vi "G#Object_GetAggregatedObjects.vi"(0 "reference in":refnum<class "G#Object.lvclass">, 2 "class attributes (F)":bool, 3 "array names (T)":bool=TRUE, 4 "remove duplicates (F)":bool, 5 "error in (no error)":errorcluster) -> (14 "reference out":refnum<class "G#Object.lvclass">, 15 "aggregated objects":refnum<class "G#Object.lvclass">[](array[class]), 16 "aggregated names":string[](array[string]), 19 "error out":errorcluster)   [LabVIEW 2020, in "G#Object.lvclass"]
doc: "Returns the aggregated objects (references in the object attributes) for the specified objects."
uses:
  <vilib>/addons/_AddQ/G#Object/G#Object.lvclass
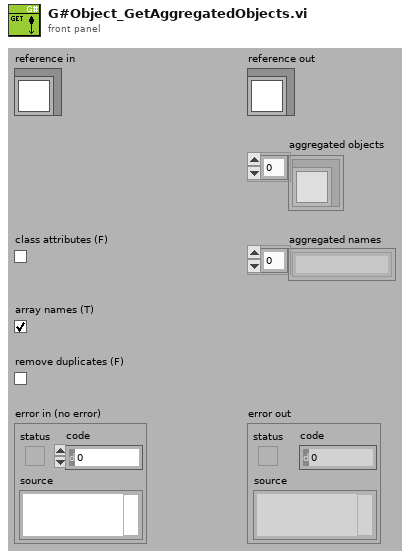
[diagram p1: front panel]
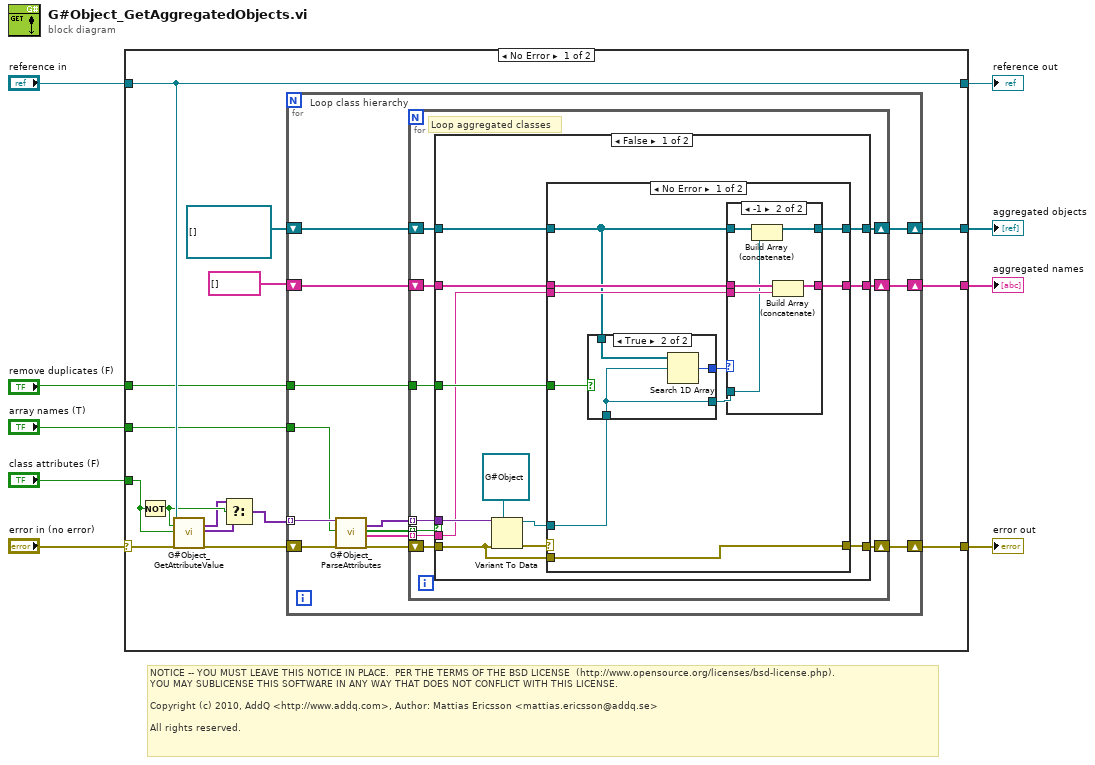
[diagram p0: block diagram]
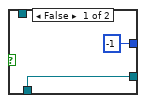
[diagram p2: hidden frame]
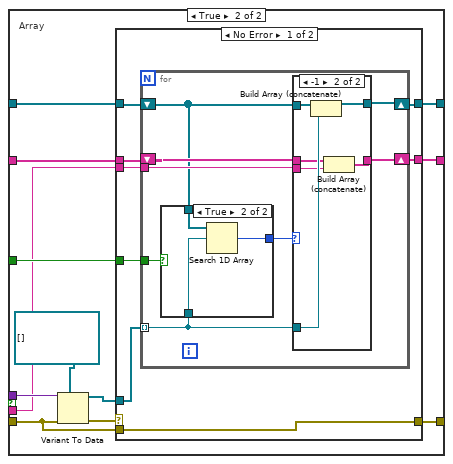
[diagram p5: hidden frame]
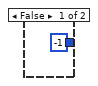
[diagram p6: hidden frame]
diagram:
  # "NOTICE -- YOU MUST LEAVE THIS NOTICE IN PLACE.  PER THE TERMS OF THE BSD LICENSE  (http://www.opensource.org/licenses/bsd-license.php).\nYOU MAY SUBLICENSE THIS SOFTWARE IN ANY WAY THAT DOES NOT CONFLICT WITH THIS LICENSE.\n\nCopyright (c) 2010, AddQ <http://www.addq.com>, Author: Mattias Ericsson <mattias.ericsson@addq.se>\n\nAll rights reserved."
  n1 = case shown="No Error" "error in (no error)" {
    selector: "error in (no error)" -> [w24 w130]
    tunnel: [w20 w130] -> w8
    tunnel: [w23 w129] -> w6
    tunnel: "reference in" -> [w23 w129]
    tunnel: [w19 _] -> w5
    tunnel: "class attributes (F)" -> [w18 _]
    tunnel: "remove duplicates (F)" -> [w13 _]
    tunnel: [w11 _] -> w2
    tunnel: "array names (T)" -> [w10 _]
    frame No Error {
      n2 = Not(x=w18) -> (.not. x?=w17:bool)
      n3 = call <vilib>:"G#Object_GetAttributeValue.vi"("reference in"=w23, "object attributes (T)"=w17, "class attributes (F)"=w18, "error in (no error)"=w24) -> ("attributes"=w16:variant[], "class attributes"=w15:variant[], "error out"=w22:errorcluster)  [unwired: 11 in, 2 out]
      n4 = Select(t=w16, s=w17, f=w15) -> (s? t:f=w14:variant[])
      n5 = for {
        shift-right: [w31] -> w20
        shift-left: w22 -> [w37]
        tunnel: w14 -> [w29] mode=indexing
        shift-right: [w32] -> w19
        shift-left: refnum<class "G#Object.lvclass">[] [] ("aggregated objects") -> [w33]
        tunnel: w13 -> [w30]
        shift-right: [w26] -> w11
        shift-left: string[] [] ("AttributeName") -> [w28]
        tunnel: w10 -> [w25]
        # "Loop class hierarchy"
        n6 = call <vilib>:"G#Object_ParseAttributes.vi"("attributes"=w29, "array names (T)"=w25, "error in (no error)"=w37) -> ("LabVIEWClassElements"=w35:variant[], "array?"=w34:bool[], "attribute name"=w27:string[], "error out"=w36:errorcluster)  [unwired: 13 in]
        n7 = for {
          shift-right: [w42] -> w31
          shift-left: w36 -> [w46]
          tunnel: w35 -> [w45] mode=indexing
          tunnel: w34 -> [w47] mode=indexing
          shift-right: [w43] -> w32
          shift-left: w33 -> [w44]
          tunnel: w30 -> [w41]
          shift-right: [w38] -> w26
          shift-left: w28 -> [w40]
          tunnel: w27 -> [w39] mode=indexing
          # "Loop aggregated classes"
          n8 = case shown="False" w47 {
            tunnel: w46 -> [w52 w91]
            tunnel: w45 -> [w59 w97]
            tunnel: w44 -> [w56 w95]
            tunnel: [w54 w94] -> w42
            tunnel: [w53 w93] -> w43
            tunnel: w41 -> [w51 w89]
            tunnel: w40 -> [w50 w88]
            tunnel: w39 -> [w49 w86]
            tunnel: [w48 w87] -> w38
            frame False {
              n9 = Variant To Data(error in=w52, type=refnum<class "G#Object.lvclass"> refnum ("G#Object.lvclass"), Variant=w59) -> (data=w55:refnum<class "G#Object.lvclass">, error out=w57:errorcluster)
              n10 = case shown="No Error" w57 {
                tunnel: w56 -> [w61 w85]
                tunnel: w55 -> [w67 _]
                tunnel: [w68 w84] -> w54
                tunnel: [w69 w85] -> w53
                tunnel: w52 -> [w68 w84]
                tunnel: w51 -> [w65 _]
                tunnel: w50 -> [w64 w83]
                tunnel: w49 -> [w63 _]
                tunnel: [w62 w83] -> w48
                frame No Error {
                  n11 = case shown="True" w65 {
                    tunnel: w67 -> [w70 w72]
                    tunnel: [-1 ("index of element") w74] -> w66
                    tunnel: w61 -> [_ w73]
                    tunnel: [w70 w72] -> w60
                    frame False {
                    }
                    frame True {
                      n12 = Search 1D Array(1D array=w73, element=w72) -> (index of element=w74:i32)  [unwired: 1 in]
                    }
                  }
                  n13 = case shown="-1" w66 {
                    tunnel: w61 -> [w76 w82]
                    tunnel: [w76 w81] -> w69
                    tunnel: w64 -> [w75 w80]
                    tunnel: w63 -> [_ w79]
                    tunnel: [w75 w78] -> w62
                    tunnel: w60 -> [_ w77]
                    frame Default {
                      # "Already\nadded"
                    }
                    frame -1 {
                      n14 = Build Array (concatenate)(w82, w77) -> (w81:refnum<class "G#Object.lvclass">[])
                      n15 = Build Array (concatenate)(w80, w79) -> (w78:string[])
                    }
                  }
                }
                frame Error {
                  # "Not a G# Object"
                }
              }
            }
            frame True {
              # "Array"
              n16 = Variant To Data(error in=w91, type=refnum<class "G#Object.lvclass">[] [] ("aggregated objects"), Variant=w97) -> (data=w90:refnum<class "G#Object.lvclass">[], error out=w96:errorcluster)
              n17 = case shown="No Error" w96 {
                tunnel: w95 -> [w104 w128]
                tunnel: [w105 w127] -> w94
                tunnel: [w103 w128] -> w93
                tunnel: w91 -> [w105 w127]
                tunnel: w90 -> [w102 _]
                tunnel: w89 -> [w101 _]
                tunnel: w88 -> [w100 w126]
                tunnel: [w99 w126] -> w87
                tunnel: w86 -> [w98 _]
                frame No Error {
                  n18 = for {
                    shift-right: [w111] -> w103
                    shift-left: w104 -> [w106]
                    tunnel: w102 -> [w112] mode=indexing
                    tunnel: w101 -> [w110]
                    shift-right: [w108] -> w99
                    shift-left: w100 -> [w109]
                    tunnel: w98 -> [w107]
                    n19 = case shown="True" w110 {
                      tunnel: [-1 ("index of element") w117] -> w113
                      tunnel: w112 -> [_ w115]
                      tunnel: w106 -> [_ w116]
                      frame False {
                      }
                      frame True {
                        n20 = Search 1D Array(1D array=w116, element=w115) -> (index of element=w117:i32)  [unwired: 1 in]
                      }
                    }
                    n21 = case shown="-1" w113 {
                      tunnel: w106 -> [w119 w125]
                      tunnel: w112 -> [_ w123]
                      tunnel: [w119 w124] -> w111
                      tunnel: w109 -> [w118 w121]
                      tunnel: [w118 w122] -> w108
                      tunnel: w107 -> [_ w120]
                      frame Default {
                        # "Already\nadded"
                      }
                      frame -1 {
                        n22 = Build Array (concatenate)(w125, w123) -> (w124:refnum<class "G#Object.lvclass">[])
                        n23 = Build Array (concatenate)(w121, w120) -> (w122:string[])
                      }
                    }
                  }
                }
                frame Error {
                  # "Not a G# Object"
                }
              }
            }
          }
        }
      }
    }
    frame Error {
    }
  }
  "error out" <- w8
  "reference out" <- w6
  "aggregated objects" <- w5
  "aggregated names" <- w2
